vi "PSVCH_Refresh VCH Formula.vi"(8 "error in":errorcluster, 9 "Formula In":string, 10 "String":string, 11 "Ref.Formula":refnum<vi>) -> (0 "error out":errorcluster, 2 "result string":string)   [LabVIEW 2016]
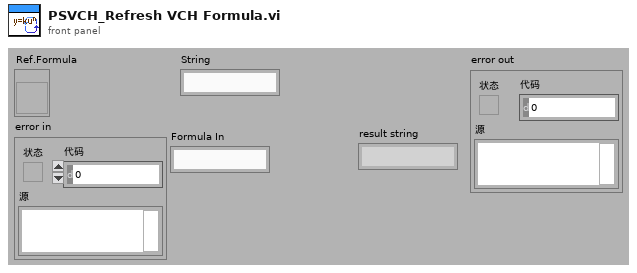
[diagram p1: front panel]
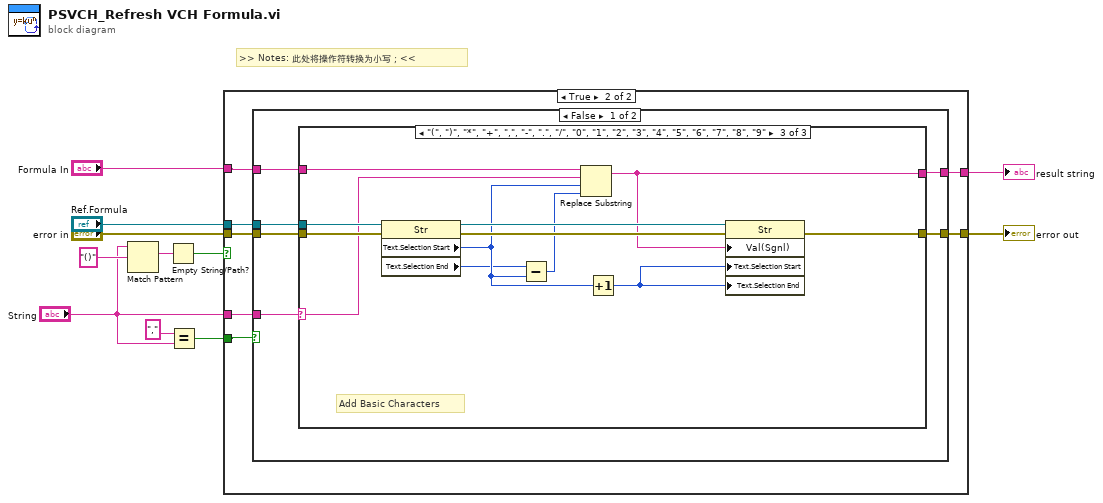
[diagram p0: block diagram]
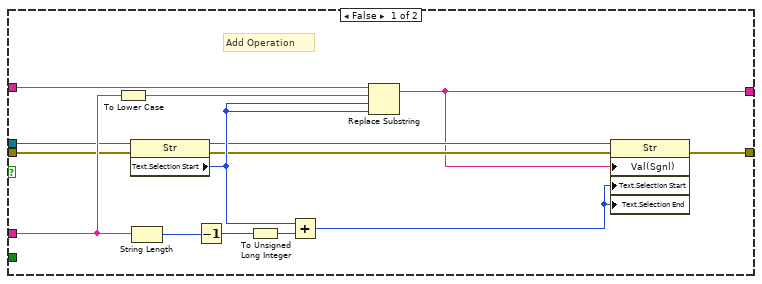
[diagram p2: hidden frame]
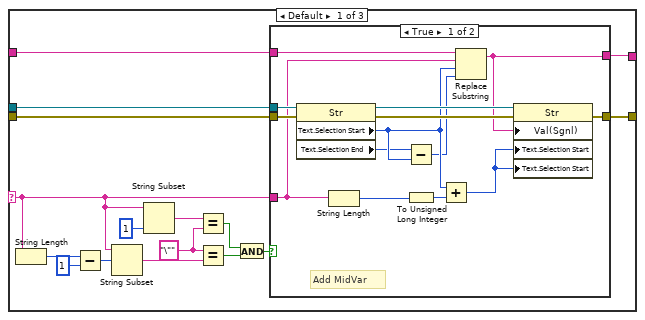
[diagram p3: hidden frame]
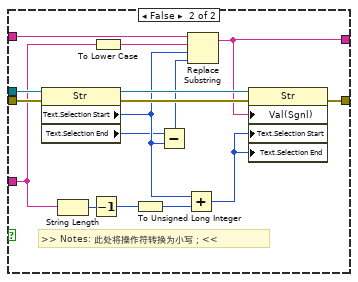
[diagram p4: hidden frame]
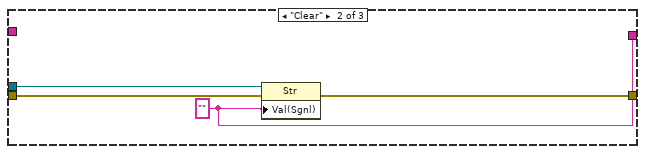
[diagram p5: hidden frame]
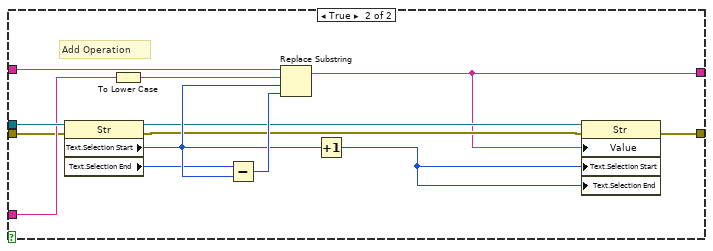
[diagram p6: hidden frame]
diagram:
  # ">> Notes: 此处将操作符转换为小写；<<"
  n1 = Match Pattern(string="String", regular expression="()" ("正则表达式")) -> (match substring=w6:string)  [unwired: 1 in, 3 out]
  n2 = Empty String/Path?(string/path=w6) -> (empty?=w3:bool)
  n3 = Equal?(x=",", y="String") -> (x = y?=w10:bool)
  n4 = case shown="True" w3 {
    tunnel: w10 -> [_ w32]
    tunnel: "Ref.Formula" -> [w18 w31]
    tunnel: [w14 w30] -> w8
    tunnel: "error in" -> [w19 w29]
    tunnel: "String" -> [w21 w28]
    tunnel: [w13 w27] -> w2
    tunnel: "Formula In" -> [w22 w26]
    frame False {
      # "Add Operation"
      n5 = To Lower Case(string=w21) -> (all lower case string=w20:string)
      n6 = property class="Str"(reference=w18, error in=w19) -> (reference out=w16:refnum<vi>, error out=w15:errorcluster, "Text.Selection Start"=w17:u32)
      n7 = String Length(string=w21) -> (length=w25:i32)
      n8 = Decrement(x=w25) -> (x-1=w24:i32)
      n9 = To Unsigned Long Integer(number=w24) -> (unsigned 32bit integer=w23:u32)
      n10 = Add(x=w17, y=w23) -> (x+y=w12:u32)
      n11 = Replace Substring(2:w17, 3:w17, 4:w20, 5:w22) -> (1:w13:string)  [unwired: 1 out]
      n12 = property class="Str"(reference=w16, error in=w15, "Val(Sgnl)"=w13, "Text.Selection Start"=w12, "Text.Selection End"=w12) -> (error out=w14:errorcluster)  [unwired: 1 out]
    }
    frame True {
      n13 = case shown="False" w32 {
        tunnel: w29 -> [w38 w108]
        tunnel: w31 -> [w37 w113]
        tunnel: w28 -> [w36 w110]
        tunnel: [w35 w103] -> w30
        tunnel: [w34 w102] -> w27
        tunnel: w26 -> [w33 w112]
        frame False {
          n14 = case shown="\"(\", \")\", \"*\", \"+\", \",\", \"-\", \".\", \"/\", \"0\", \"1\", \"2\", \"3\", \"4\", \"5\", \"6\", \"7\", \"8\", \"9\"" w36 {
            selector: w36 -> [w42 _ w92]
            tunnel: w38 -> [w44 w88 w100]
            tunnel: w37 -> [w43 w87 w99]
            tunnel: [w41 w86 w96] -> w35
            tunnel: [w40 w85 w90] -> w34
            tunnel: w33 -> [w39 _ w95]
            frame Default {
              w48 = "\""
              n15 = String Length(string=w42) -> (length=w53:i32)
              n16 = Subtract(x=w53, y=1) -> (x-y=w52:i32)
              n17 = String Subset(string=w42, offset (0)=w52) -> (substring=w50:string)  [unwired: 1 in]
              n18 = String Subset(string=w42, length (rest)=1 ("length (rest)")) -> (substring=w49:string)  [unwired: 1 in]
              n19 = Equal?(x=w49, y=w48) -> (x = y?=w47:bool)
              n20 = Equal?(x=w48, y=w50) -> (x = y?=w46:bool)
              n21 = And(x=w47, y=w46) -> (x .and. y?=w45:bool)
              n22 = case shown="True" w45 {
                tunnel: w44 -> [w65 w81]
                tunnel: w43 -> [w64 w80]
                tunnel: w42 -> [w58 w73]
                tunnel: [w62 w78] -> w41
                tunnel: [w56 w70] -> w40
                tunnel: w39 -> [w61 w76]
                frame True {
                  # "Add MidVar"
                  n23 = property class="Str"(reference=w64, error in=w65) -> (reference out=w67:refnum<vi>, error out=w66:errorcluster, "Text.Selection Start"=w60:u32, "Text.Selection End"=w57:u32)
                  n24 = String Length(string=w58) -> (length=w63:i32)
                  n25 = Subtract(x=w57, y=w60) -> (x-y=w59:u32)
                  n26 = To Unsigned Long Integer(number=w63) -> (unsigned 32bit integer=w68:u32)
                  n27 = Add(x=w60, y=w68) -> (x+y=w55:u32)
                  n28 = Replace Substring(2:w59, 3:w60, 4:w58, 5:w61) -> (1:w56:string)  [unwired: 1 out]
                  n29 = property class="Str"(reference=w67, error in=w66, "Val(Sgnl)"=w56, "Text.Selection Start"=w55, "Text.Selection Start"=w55) -> (error out=w62:errorcluster)  [unwired: 1 out]
                }
                frame False {
                  # ">> Notes: 此处将操作符转换为小写；<<"
                  n30 = property class="Str"(reference=w80, error in=w81) -> (reference out=w83:refnum<vi>, error out=w82:errorcluster, "Text.Selection Start"=w75:u32, "Text.Selection End"=w71:u32)
                  n31 = String Length(string=w73) -> (length=w79:i32)
                  n32 = Decrement(x=w79) -> (x-1=w77:i32)
                  n33 = To Lower Case(string=w73) -> (all lower case string=w72:string)
                  n34 = To Unsigned Long Integer(number=w77) -> (unsigned 32bit integer=w84:u32)
                  n35 = Subtract(x=w71, y=w75) -> (x-y=w74:u32)
                  n36 = Add(x=w75, y=w84) -> (x+y=w69:u32)
                  n37 = Replace Substring(2:w74, 3:w75, 4:w72, 5:w76) -> (1:w70:string)  [unwired: 1 out]
                  n38 = property class="Str"(reference=w83, error in=w82, "Val(Sgnl)"=w70, "Text.Selection Start"=w69, "Text.Selection End"=w69) -> (error out=w78:errorcluster)  [unwired: 1 out]
                }
              }
            }
            frame "Clear" {
              w85 = "" ("Value")
              n39 = property class="Str"(reference=w87, error in=w88, "Val(Sgnl)"=w85) -> (error out=w86:errorcluster)  [unwired: 1 out]
            }
            frame "(", ")", "*", "+", ",", "-", ".", "/", "0", "1", "2", "3", "4", "5", "6", "7", "8", "9" {
              # "Add Basic Characters"
              n40 = property class="Str"(reference=w99, error in=w100) -> (reference out=w97:refnum<vi>, error out=w98:errorcluster, "Text.Selection Start"=w94:u32, "Text.Selection End"=w91:u32)
              n41 = Subtract(x=w91, y=w94) -> (x-y=w93:u32)
              n42 = Replace Substring(2:w93, 3:w94, 4:w92, 5:w95) -> (1:w90:string)  [unwired: 1 out]
              n43 = Increment(x=w94) -> (x+1=w89:u32)
              n44 = property class="Str"(reference=w97, error in=w98, "Val(Sgnl)"=w90, "Text.Selection Start"=w89, "Text.Selection End"=w89) -> (error out=w96:errorcluster)  [unwired: 1 out]
            }
          }
        }
        frame True {
          # "Add Operation"
          n45 = property class="Str"(reference=w113, error in=w108) -> (reference out=w105:refnum<vi>, error out=w104:errorcluster, "Text.Selection Start"=w107:u32, "Text.Selection End"=w106:u32)
          n46 = To Lower Case(string=w110) -> (all lower case string=w109:string)
          n47 = Subtract(x=w106, y=w107) -> (x-y=w111:u32)
          n48 = Replace Substring(2:w111, 3:w107, 4:w109, 5:w112) -> (1:w102:string)  [unwired: 1 out]
          n49 = Increment(x=w107) -> (x+1=w101:u32)
          n50 = property class="Str"(reference=w105, error in=w104, "Value"=w102, "Text.Selection Start"=w101, "Text.Selection End"=w101) -> (error out=w103:errorcluster)  [unwired: 1 out]
        }
      }
    }
  }
  "error out" <- w8
  "result string" <- w2
